vi "Software Update HCC Create Archive Folder.vi"(6 "Station Location (Index)":u32, 8 "error in (no error)":errorcluster, 9 "Newfi Exe Folder Path":path=path "C:/Newfi Exe", 10 "Path":path, 11 "folder names":string[](array[string])) -> (0 "error out":errorcluster, 2 "Output Path Archive Folder":path)   [LabVIEW 2016]
panel:
  out "Configuration File":string[][](array[string])
  out "List of Stations and Board IDs":string[][](array[string])
  out "Updated Configuration File":string[][](array[string])
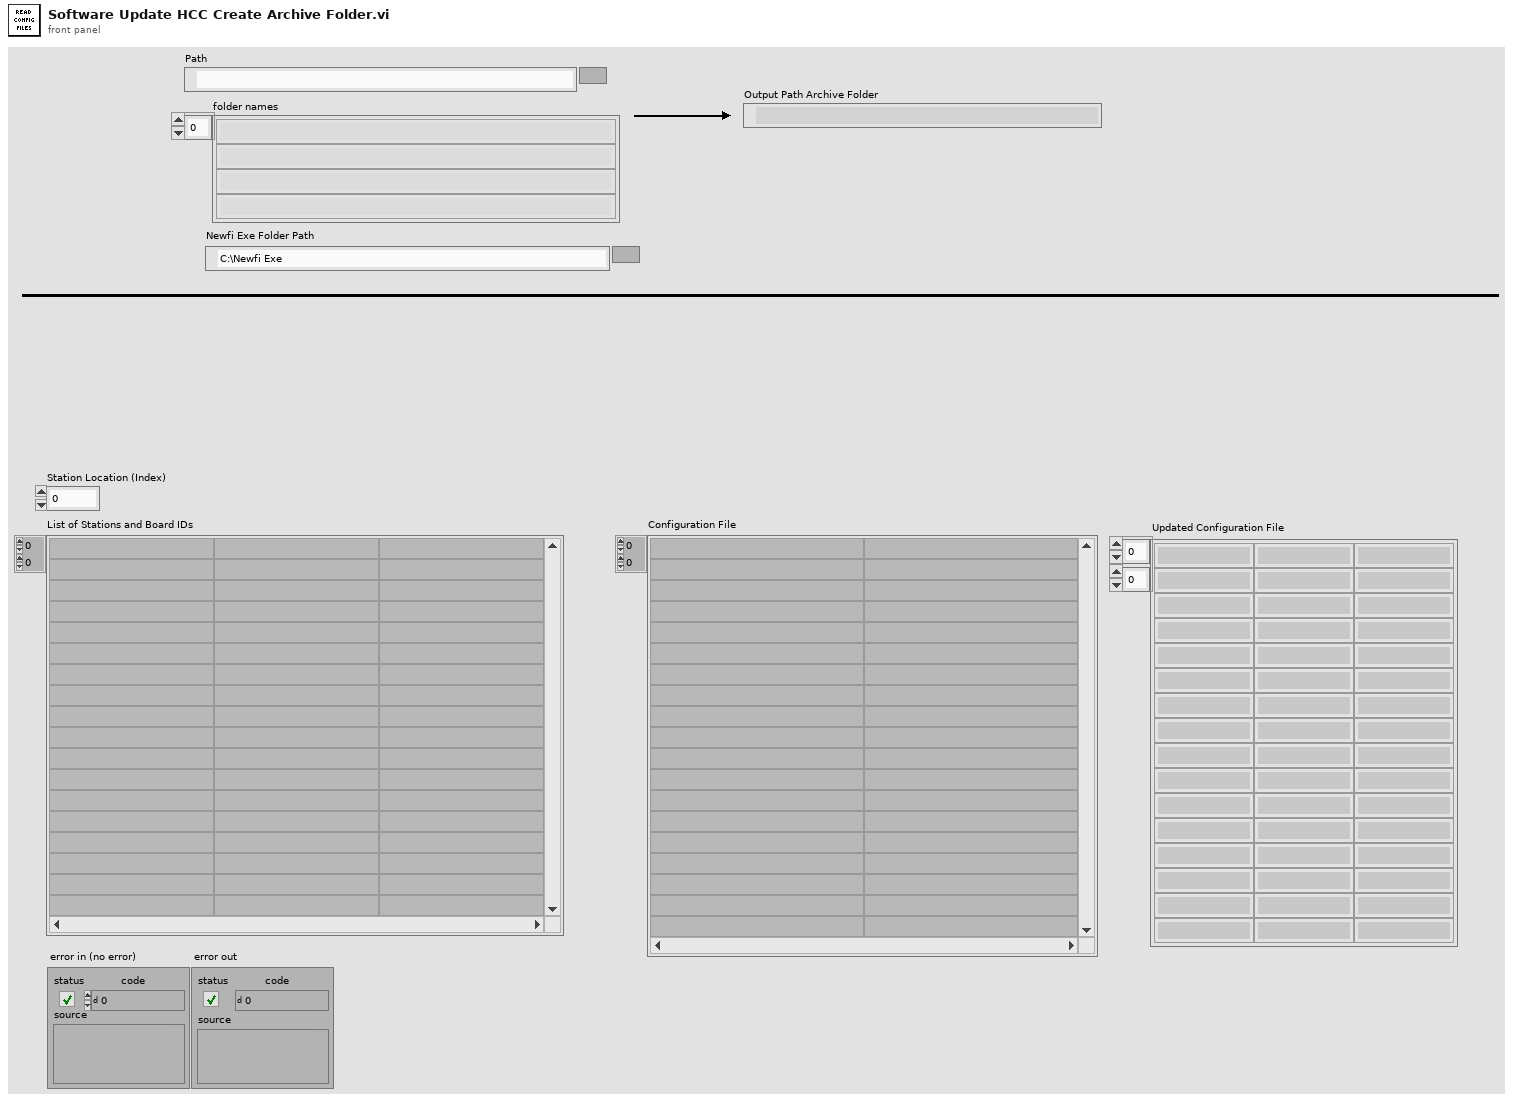
[diagram p1: front panel]
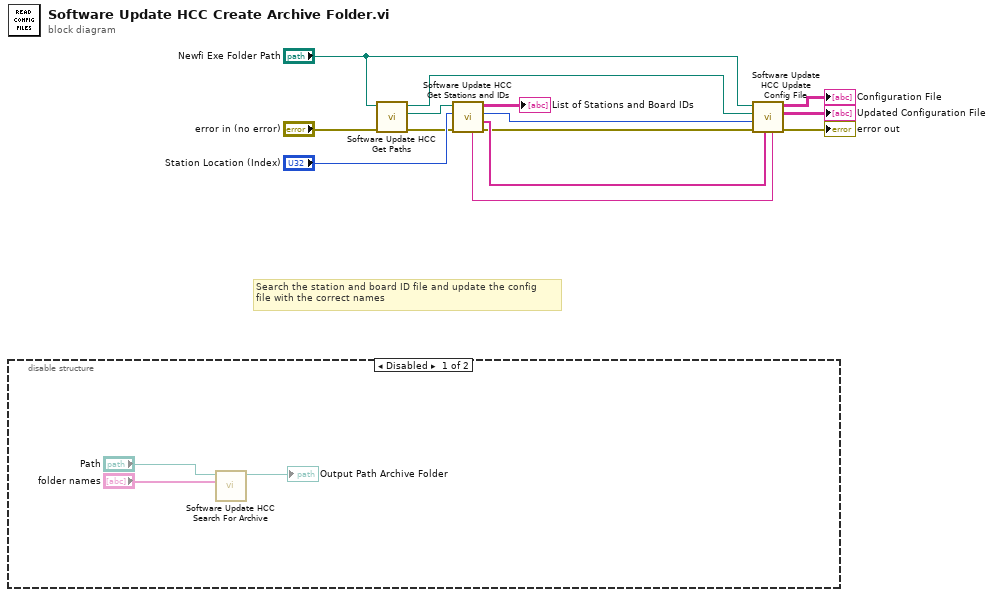
[diagram p0: block diagram]
diagram:
  # "Search the station and board ID file and update the config\nfile with the correct names"
  n1 = disable-structure shown="Disabled" {
    frame Disabled {
      n2 = call "Software Update HCC Search For Archive.vi"("folder names"="folder names", "Path"="Path") -> ("error out"=w18:errorcluster, "Output Path Archive Folder"=→"Output Path Archive Folder":path)  [unwired: 8 in]
    }
    frame Enabled {
    }
  }
  n3 = call "Software Update HCC Get Paths.vi"("Error In"="error in (no error)", "Newfi Exe Folder Path"="Newfi Exe Folder Path") -> ("Error Out"=w5:errorcluster, "Stations and Board IDs"=w10:path, "Newfi Exe Locations"=w11:path)  [unwired: 7 in]
  n4 = call "Software Update HCC Get Stations and IDs.vi"("Error In"=w5, "Station Location (Index)"="Station Location (Index)", "Stations and Board IDs"=w10) -> ("Error Out"=w6:errorcluster, "Updated Input"=w14:string[], "Station index"=w12:u32, "List of Stations and Board IDs"=→"List of Stations and Board IDs":string[][], "Station Name"=w4:string)  [unwired: 4 in]
  n5 = call "Software Update HCC Update Config File.vi"("Station Name"=w4, "Updated Input"=w14, "Error In"=w6, "Station index"=w12, "Newfi Exe Locations"=w11, "Newfi Exe Folder Path"="Newfi Exe Folder Path") -> ("Error Out"=→"error out":errorcluster, "Updated Configuration File"=→"Updated Configuration File":string[][], "Configuration File"=→"Configuration File":string[][])  [unwired: 3 in]
